vi "Parametros.vi"(0 "VetorDeDados":dbl[][](array[numeric]), 11 "pontos":dbl) -> (4 "Icc":dbl, 6 "Vca":dbl, 8 "Pmp":dbl, 10 "Vmp":dbl, 15 "Imp":dbl)   [LabVIEW 2012]
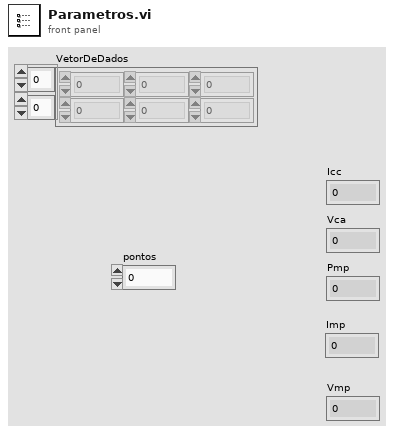
[diagram p1: front panel]
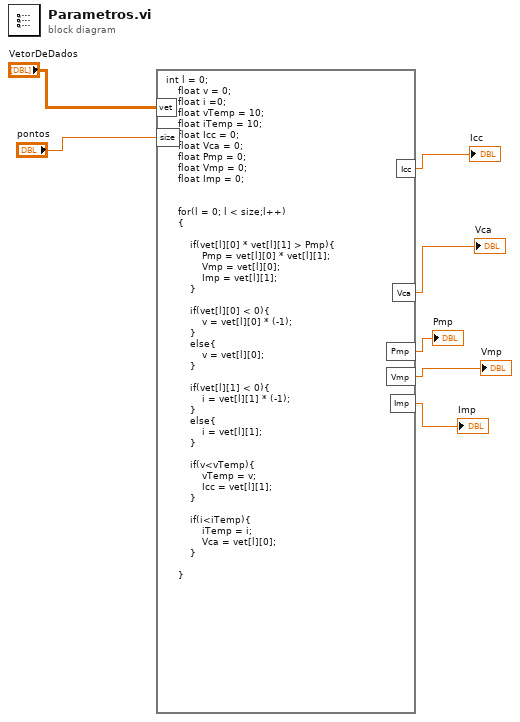
[diagram p0: block diagram]
diagram:
  n1 = formula code="int l = 0;\n    float v = 0;\n    float i =0;\n    float vTemp = 10;\n    float iTemp = 10;\n    float Icc = 0;\n    float Vca = 0;\n    float Pmp = 0;\n    float Vmp = 0;\n    float Imp = 0;\n\n\n    for(l = 0; l < size;l++)\n    {\n    \n        if(vet[l][0] * vet[l][1] > Pmp){\n            Pmp = vet[l][0] * vet[l][1];\n            Vmp = vet[l][0];\n            Imp = vet[l][1];\n        }\n\n        if(vet[l][0] < 0){\n            v = vet[l][0] * (-1);\n        }\n        else{\n            v = vet[l][0];\n        }\n\n        if(vet[l][1] < 0){\n            i = vet[l][1] * (-1);\n        }\n        else{\n            i = vet[l][1];\n        }\n\n        if(v<vTemp){\n            vTemp = v;\n            Icc = vet[l][1];\n        }\n\n        if(i<iTemp){\n            iTemp = i;\n            Vca = vet[l][0];\n        }\n\n    }"("vet"="VetorDeDados", "size"="pontos") -> ("Icc"=→"Icc":dbl, "Vca"=→"Vca":dbl, "Pmp"=→"Pmp":dbl, "Imp"=→"Imp":dbl, "Vmp"=→"Vmp":dbl)
